vi "HapticSTM_write_test-bench.vi"() -> ()   [LabVIEW 2019]
uses:
  SubVIs/GlobalClicksHeight.vi
  <userlib>/HapticSTM/HapticSTM.lvlib
panel:
  out "Safetip":bool
  out "Forces":cluster{"Fy":dbl, "Fz":dbl, "Fx":dbl} {"Fy" format="%.1f"; "Fz" format="%.1f"; "Fx" format="%.1f"}
  out "Position":cluster{"X":dbl, "Y":dbl, "Z pen":dbl, "Z":dbl}
  out "Frame Properties":cluster{"Ox":dbl, "Oy":dbl, "Fw":dbl, "Fh":dbl}
  in  "XY Write?":bool=TRUE
  in  "Z Write?":bool
  in  "Save":bool
  in  "# Sample Points":i32=4096
  in  "Depth (pA)":dbl=280.0
  in  "Shift (in)":dbl format="%.1f"
  in  "Hardness":dbl=0.7 format="%.1f"
  in  "Scaling?":u16(ring) items=["Medium", "Large", "Small"]
  out "Setpoint (pA)":dbl
  in  "Maximum (pA)":dbl=7000.0
  out "Filtered Current (pA)":dbl format="%.1f"
  out "Current (pA)":dbl format="%.1f"
  out "Z Write":dbl format="%^.1e"
  in  "Planing?":bool
  in  "Mode":u16(ring) items=["Log w/ Exp Z", "Log w/ Lin Z", "Coulomb Force", "Lennard Jones", "r^6"]
  in  "Reset Clicks":bool
  out "Clicks":i32
  in  "STOP":bool
  in  "START":bool
  # "Super Ultra Mega Haptic STM Controller 3000"
  # "Haptic Pen"
  # "Nanonis"
  # "Position"
  # "Z Controller"
  # "Force"
  # "Frame"
  # "Surface"
  # "Options"
  # "Current"
  # "No"
  # "Yes"
  # "Planing"
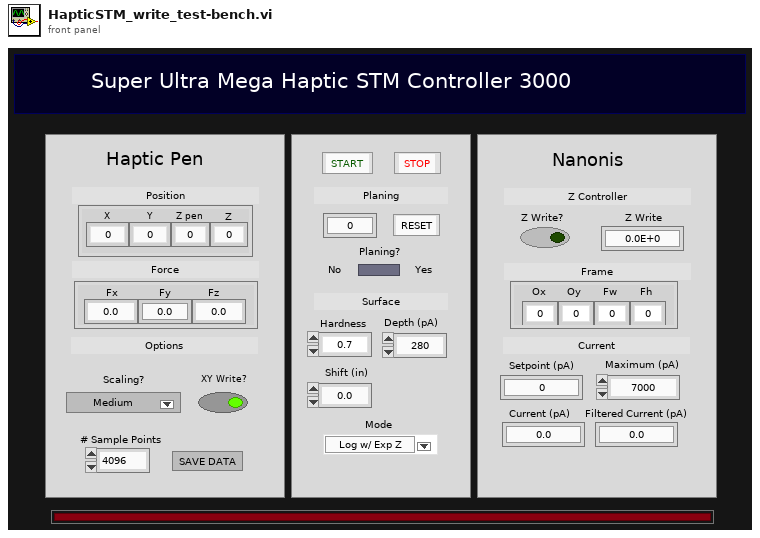
[diagram p1: front panel]
types:
  T1 = cluster{"X Origin (nm)":dbl, "Y Origin (nm)":dbl, "FW (nm)":dbl, "FH (nm)":dbl}
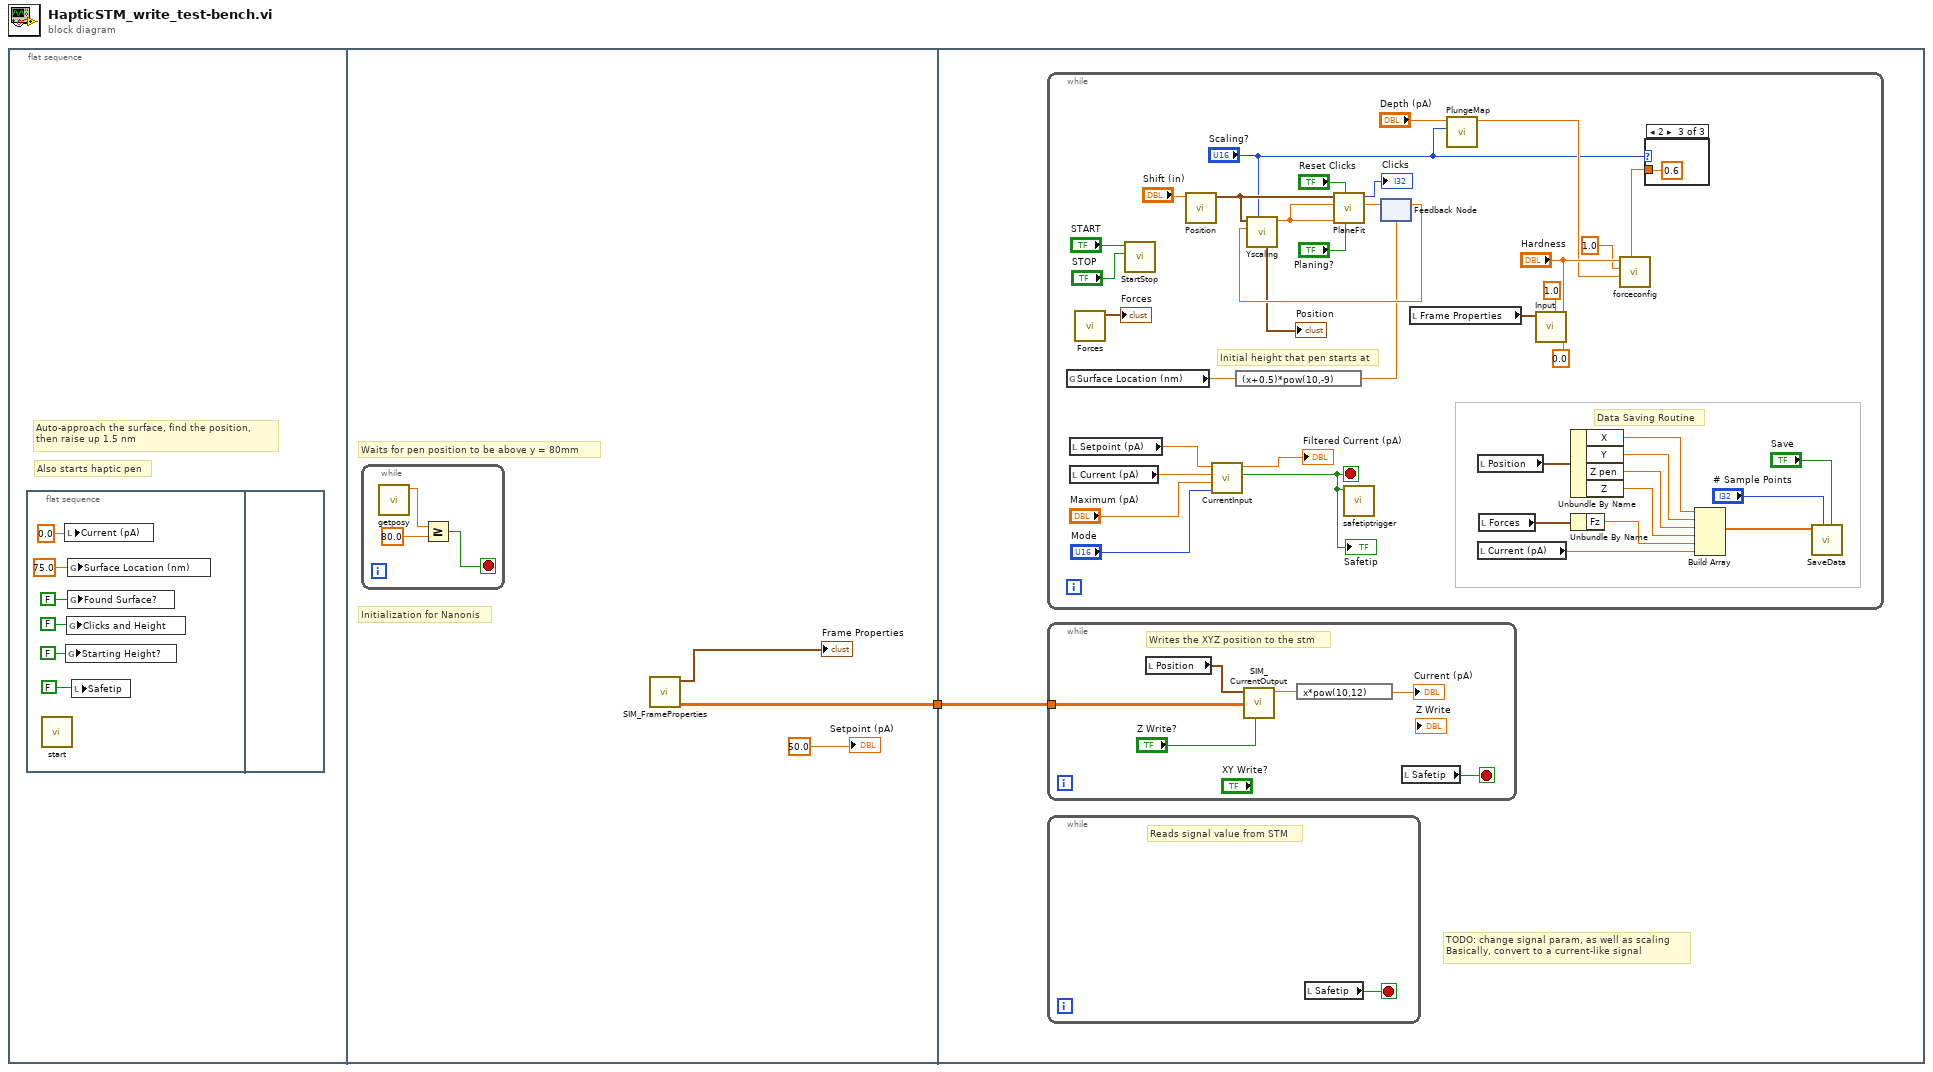
[diagram p0: block diagram]
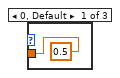
[diagram p2: hidden frame]
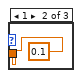
[diagram p3: hidden frame]
diagram:
  n1 = flat-sequence {
    tunnel: [w8] -> w1
    tunnel: w1 -> [w14]
    frame #0 {
      # "Also starts haptic pen"
      # "Auto-approach the surface, find the position, \nthen raise up 1.5 nm"
      n2 = flat-sequence {
        frame #0 {
          n3 = call <userlib>:"start.vi"() -> ()  [unwired: 11 in, 1 out]
          n4 = local write "Current (pA)"(0.0 ("Current (pA)")) -> ()
          n5 = global write "GlobalClicksHeight.vi" "Starting Height?"(FALSE ("Clicks and Height")) -> ()
          n6 = global write "GlobalClicksHeight.vi" "Clicks and Height"(FALSE ("Clicks and Height")) -> ()
          n7 = global write "GlobalClicksHeight.vi" "Surface Location (nm)"(75.0 ("Surface Location")) -> ()
          n8 = global write "GlobalClicksHeight.vi" "Found Surface?"(FALSE ("Clicks and Height")) -> ()
          n9 = local write "Safetip"(FALSE ("Safe Tip?")) -> ()
        }
        frame #1 {
        }
      }
    }
    frame #1 {
      # "Waits for pen position to be above y = 80mm"
      # "Initialization for Nanonis"
      n10 = while {
        stop <- w11 stop-if-true
        n11 = call <userlib>:"getposy.vi"() -> ("function return"=w13:dbl)  [unwired: 11 in]
        n12 = Greater Or Equal?(x=w13, y=80.0) -> (x >= y?=w11:bool)
      }
      n13 = call "SIM_FrameProperties.vi"() -> ("data"=w8:dbl[][], "Frame Properties"=→"Frame Properties":T1)  [unwired: 10 in]
      "Setpoint (pA)" <- 50.0 ("Setpoint (pA)")
    }
    frame #2 {
      # "TODO: change signal param, as well as scaling\nBasically, convert to a current-like signal"
      n14 = while {
        stop <- w22 stop-if-true
        # "Data Saving Routine"
        # "Initial height that pen starts at"
        n15 = global read "GlobalClicksHeight.vi" "Surface Location (nm)"() -> (w33:dbl)
        n16 = local read "Setpoint (pA)"() -> (w31:dbl)
        n17 = local read "Current (pA)"() -> (w30:dbl)
        n18 = call "Forces.vi"() -> ("Forces"=→"Forces":cluster{"Fy":dbl, "Fz":dbl, "Fx":dbl})  [unwired: 11 in]
        n19 = call "StartStop.vi"("STOP"="STOP", "START"="START") -> ()  [unwired: 10 in]
        n20 = call "Position.vi"("Shift"="Shift (in)") -> ("Position"=w40:cluster{"X":dbl, "Y":dbl, "Zpen":dbl})  [unwired: 10 in]
        n21 = call "CurrentInput.vi"("Mode"="Mode", "Maximum (pA)"="Maximum (pA)", "Current (pA)"=w30, "Setpoint (pA)"=w31) -> ("Safetip?"=w22:bool, "Filtered Current (pA)"=→"Filtered Current (pA)":dbl)  [unwired: 6 in]
        "Safetip" <- w22
        n22 = expression code="(x+0.5)*pow(10,-9)"(w33) -> (w32:dbl)
        n23 = call <userlib>:"safetiptrigger.vi"("triggered"=w22) -> ()  [unwired: 11 in]
        n24 = feedback #1(w32) -> (w42:dbl)
        n25 = call "Yscaling.vi"("Scaling?"="Scaling?", "Plane Height (m)"=w42, 11:w40) -> ("y scaled (m)"=w29:dbl, "Position"=→"Position":cluster{"X":dbl, "Y":dbl, "Z pen":dbl, "Z":dbl})  [unwired: 6 in, 1 out]
        n26 = call "PlaneFit.vi"("Planing y/n?"="Planing?", "Reset Clicks"="Reset Clicks", "Y PEN"=w29, "Nano Z"=w29, "Position"=w40) -> ("Plane Height (m)"=w55:dbl, "Clicks"=→"Clicks":i32)  [unwired: 4 in, 1 out]
        n27 = feedback-in #1(w55) -> ()
        n28 = local read "Frame Properties"() -> (w41:cluster{"Ox":dbl, "Oy":dbl, "Fw":dbl, "Fh":dbl})
        n29 = call "PlungeMap.vi"("Scaling?"="Scaling?", "Input (pA)"="Depth (pA)") -> ("output"=w28:dbl)  [unwired: 9 in]
        n30 = local read "Position"() -> (w38:cluster{"X":dbl, "Y":dbl, "Z pen":dbl, "Z":dbl})
        n31 = local read "Current (pA)"() -> (w24:dbl)
        n32 = local read "Forces"() -> (w26:cluster{"Fy":dbl, "Fz":dbl, "Fx":dbl})
        n33 = call "Input.vi"("Current * 10^input"=0.0, "Sensitivity"="Hardness", "Drag"=1.0, "Frame Properties (Remapped)"=w41) -> ()  [unwired: 6 in, 2 out]
        n34 = Unbundle By Name(w38) -> ("X"=w37:dbl, "Y"=w36:dbl, "Z pen"=w35:dbl, "Z"=w34:dbl)
        n35 = Unbundle By Name(w26) -> ("Fz"=w25:dbl)
        n36 = case shown="2" "Scaling?" {
          tunnel: [0.5 0.1 0.6] -> w45
          frame 0, Default {
          }
          frame 1 {
          }
          frame 2 {
          }
        }
        n37 = call <userlib>:"forceconfig.vi"("spc"=w45, "c"=w28, "b"=1.0, "a"="Hardness") -> ()  [unwired: 8 in]
        n38 = Build Array(w37, w36, w35, w34, w25, w24) -> (w61:dbl[])
        n39 = call "SaveData.vi"("Save"="Save", "# Sample Points"="# Sample Points", "Data"=w61) -> ()  [unwired: 9 in]
      }
      n40 = while {
        tunnel: w14 -> [w17]
        stop <- w21 stop-if-true
        # "Writes the XYZ position to the stm"
        n41 = local read "Position"() -> (w20:cluster{"X":dbl, "Y":dbl, "Z pen":dbl, "Z":dbl})
        n42 = call "SIM_CurrentOutput.vi"("Z Write?"="Z Write?", "array"=w17, "Position"=w20) -> ("Current Out (pA)"=w18:dbl)  [unwired: 8 in]
        n43 = expression code="x*pow(10,12)"(w18) -> (→"Current (pA)":dbl)
        n44 = local read "Safetip"() -> (w21:bool)
      }
      n45 = while {
        stop <- w15 stop-if-true
        # "Reads signal value from STM"
        n46 = local read "Safetip"() -> (w15:bool)
      }
    }
  }
